vi "Ex-Analysis.vi"() -> ()   [LabVIEW 2010]
doc: "Use this template to generate a signal, analyze the signal, and display the result. You can use this template with the exercises in the Getting Started with LabVIEW manual.\nNote: LabVIEW enables automatic error handling by default for VIs you create from this template."
uses:
  <vilib>/express/express arith-compare/Formula/XNode/ExpressFormulaBlockNode.xnode
  Instance           1 34Saved   TutorialGenAnalyzeDisp.vit .vi
  Instance           2 34Saved   TutorialGenAnalyzeDisp.vit .vi
  <vilib>/express/express shared/transition.llb/Dynamic To Waveform Array.vi
  <vilib>/express/express shared/transition.llb/Waveform Array To Dynamic.vi
  <vilib>/express/express arith-compare/Formula/Block/exnFormulaBlock how many pts in the wave.vi
  <vilib>/express/express shared/ex_Modify Signal Name.vi
panel:
  out "Filtered Signal":dynamicdata(graph)
  out "Unfiltered Signal":dynamicdata(graph)
  out "RMS":dbl
  in  "stop":bool
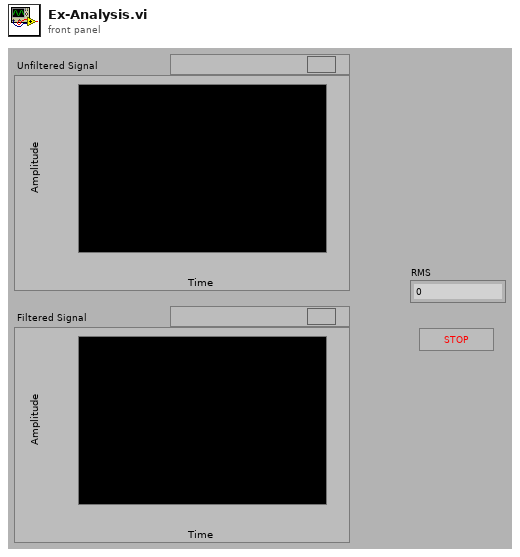
[diagram p1: front panel]
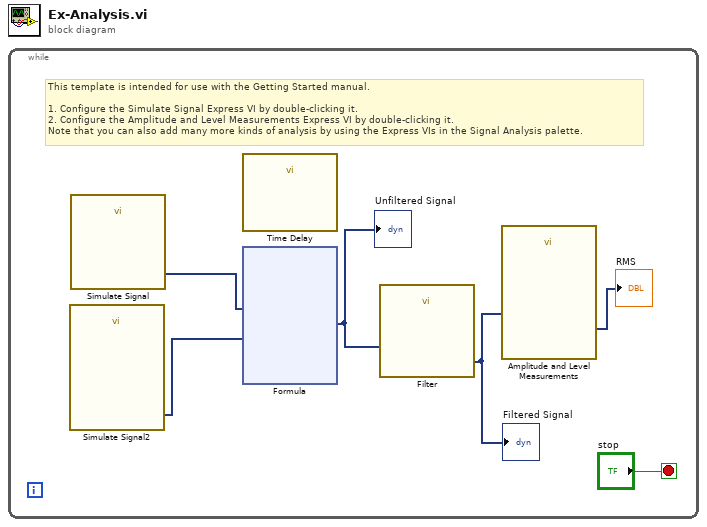
[diagram p0: block diagram]
diagram:
  n1 = while {
    stop <- "stop" stop-if-true
    # "This template is intended for use with the Getting Started manual.\n\n1. Configure the Simulate Signal Express VI by double-clicking it.\n2. Configure the Amplitude and Level Measurements Express VI by double-clicking it.\nNote that you can also add many more kinds of analysis by using the Express VIs in the Signal Analysis palette."
    n2 = call "Simulate Signal2"() -> ("60 Hz and Noise"=w3:dynamicdata)  [unwired: 14 in, 1 out]
    n3 = call "Simulate Signal"() -> ("Sine"=w4:dynamicdata)  [unwired: 14 in, 1 out]
    n4 = call "Time Delay"() -> ()  [unwired: 11 in, 1 out]
    n5 = xnode "Formula"("Sine"=w4, "60 Hz and Noise"=w3) -> ("Result"=w2:dynamicdata)  [unwired: 1 in, 1 out]
    "Unfiltered Signal" <- w2
    n6 = call "Filter"("Signal"=w2) -> ("Filtered Signal"=w1:dynamicdata)  [unwired: 9 in, 1 out]
    "Filtered Signal" <- w1
    n7 = call "Amplitude and Level Measurements"("Signals"=w1) -> ("RMS"=→"RMS":dynamicdata)  [unwired: 12 in, 2 out]
  }
